vi "sensores_andar_adq.vi"(0 "C1-J":dbl, 1 "C2-M":dbl, 2 "C2-J":dbl, 3 "C3-M":dbl, 4 "C3-J":dbl, 5 "C4-M":dbl, 6 "C1-M":dbl, 7 "C4-J":dbl, 8 "Pfundo(kPa)":dbl) -> (12 "Estação 1 W":bool, 13 "Estação 4 K":bool, 14 "Estação 1 K":bool, 15 "Estação 2 W":bool, 16 "Estação 2 K":bool, 17 "Estação 3 W":bool, 18 "Estação 3 K":bool, 19 "Estação 4 W":bool)   [LabVIEW 2019]
doc: "VI de acionamento de andares de acordo com as tensões nos sensores capacitivos, com essa VI conseguimos ver animadamente a água passando pela linha e retirando querosene ou vice versa"
panel:
  # "ESTA敲O 4"
  # "ESTA敲O 3"
  # "ESTA敲O 2"
  # "ESTA敲O 1"
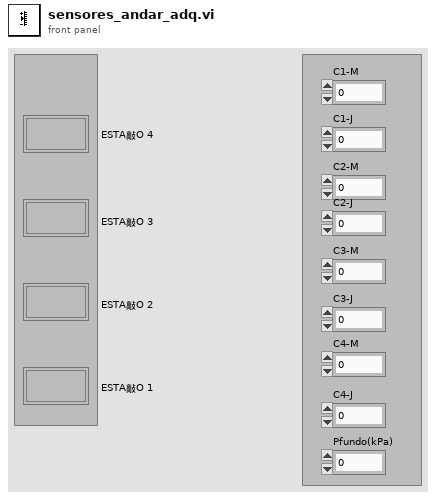
[diagram p1: front panel]
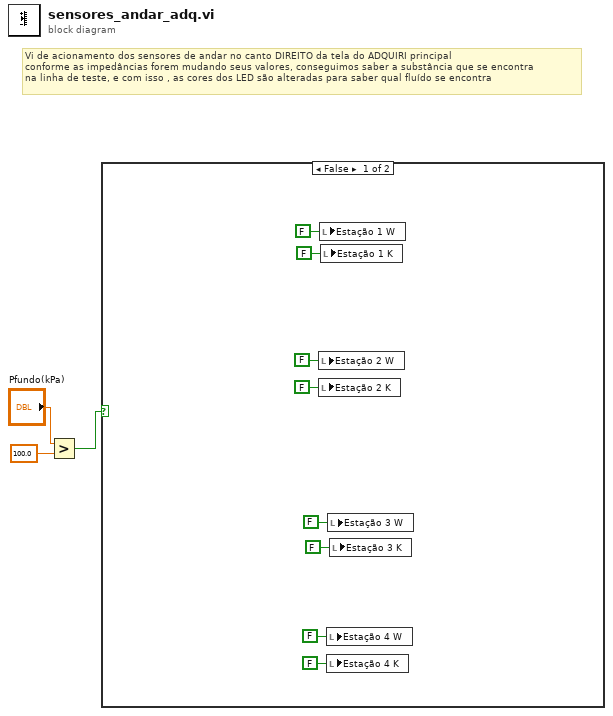
[diagram p0: block diagram]
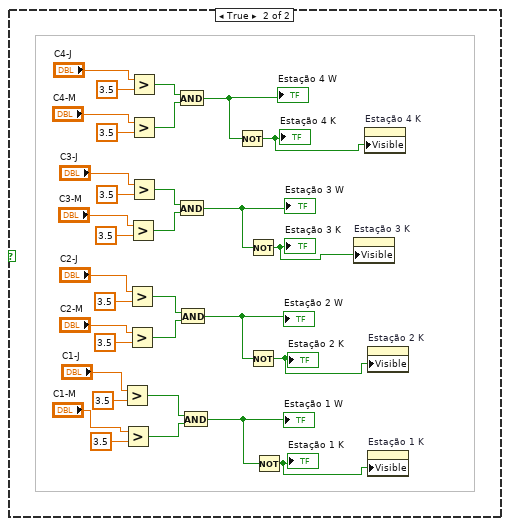
[diagram p2: hidden frame]
diagram:
  # "Vi de acionamento dos sensores de andar no canto DIREITO da tela do ADQUIRI principal\nconforme as impedâncias forem mudando seus valores, conseguimos saber a substância que se encontra\nna linha de teste, e com isso , as cores dos LED são alteradas para saber qual fluído se encontra"
  n1 = Greater?(x="Pfundo(kPa)", y=100.0) -> (0:w1:bool)
  n2 = case shown="False" w1 {
    frame False {
      n3 = local write "Estação 2 W"(FALSE ("Estação 2 W")) -> ()
      n4 = local write "Estação 2 K"(FALSE ("Estação 2 K")) -> ()
      n5 = local write "Estação 1 W"(FALSE ("Estação 1 W")) -> ()
      n6 = local write "Estação 1 K"(FALSE ("Estação 1 K")) -> ()
      n7 = local write "Estação 4 W"(FALSE ("Estação 4 W")) -> ()
      n8 = local write "Estação 4 K"(FALSE ("Estação 4 K")) -> ()
      n9 = local write "Estação 3 W"(FALSE ("Estação 3 W")) -> ()
      n10 = local write "Estação 3 K"(FALSE ("Estação 3 K")) -> ()
    }
    frame True {
      n11 = Greater?(x="C1-J", y=3.5) -> (0:w26:bool)
      n12 = Greater?(x="C1-M", y=3.5) -> (0:w27:bool)
      n13 = Greater?(x="C2-J", y=3.5) -> (0:w24:bool)
      n14 = Greater?(x="C2-M", y=3.5) -> (0:w25:bool)
      n15 = Greater?(x="C3-M", y=3.5) -> (0:w23:bool)
      n16 = Greater?(x="C4-J", y=3.5) -> (0:w20:bool)
      n17 = Greater?(x="C4-M", y=3.5) -> (0:w21:bool)
      n18 = Greater?(x="C3-J", y=3.5) -> (0:w22:bool)
      n19 = And(x=w20, y=w21) -> (x .and. y?=w16:bool)
      "Estação 4 W" <- w16
      n20 = And(x=w22, y=w23) -> (x .and. y?=w17:bool)
      "Estação 3 W" <- w17
      n21 = And(x=w24, y=w25) -> (x .and. y?=w18:bool)
      "Estação 2 W" <- w18
      n22 = And(x=w26, y=w27) -> (x .and. y?=w19:bool)
      "Estação 1 W" <- w19
      n23 = Not(x=w16) -> (.not. x?=w12:bool)
      "Estação 4 K" <- w12
      n24 = Not(x=w17) -> (.not. x?=w15:bool)
      "Estação 3 K" <- w15
      n25 = Not(x=w18) -> (.not. x?=w13:bool)
      "Estação 2 K" <- w13
      n26 = Not(x=w19) -> (.not. x?=w14:bool)
      "Estação 1 K" <- w14
      n27 = property on="Estação 3 K" class="Bool (strict)"("Visible"=w15) -> ()  [unwired: 2 in, 2 out]
      n28 = property on="Estação 4 K" class="Bool (strict)"("Visible"=w12) -> ()  [unwired: 2 in, 2 out]
      n29 = property on="Estação 2 K" class="Bool (strict)"("Visible"=w13) -> ()  [unwired: 2 in, 2 out]
      n30 = property on="Estação 1 K" class="Bool (strict)"("Visible"=w14) -> ()  [unwired: 2 in, 2 out]
    }
  }
